vi "Start_Ramping.vi"() -> (3 "Setpoint":dbl)   [LabVIEW 2016]
uses:
  Instrument_Setup.vi
  Global/Global Variables/global.vi
  Global/Global Variables/Data_Display_global.vi
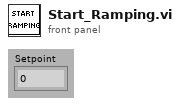
[diagram p1: front panel]
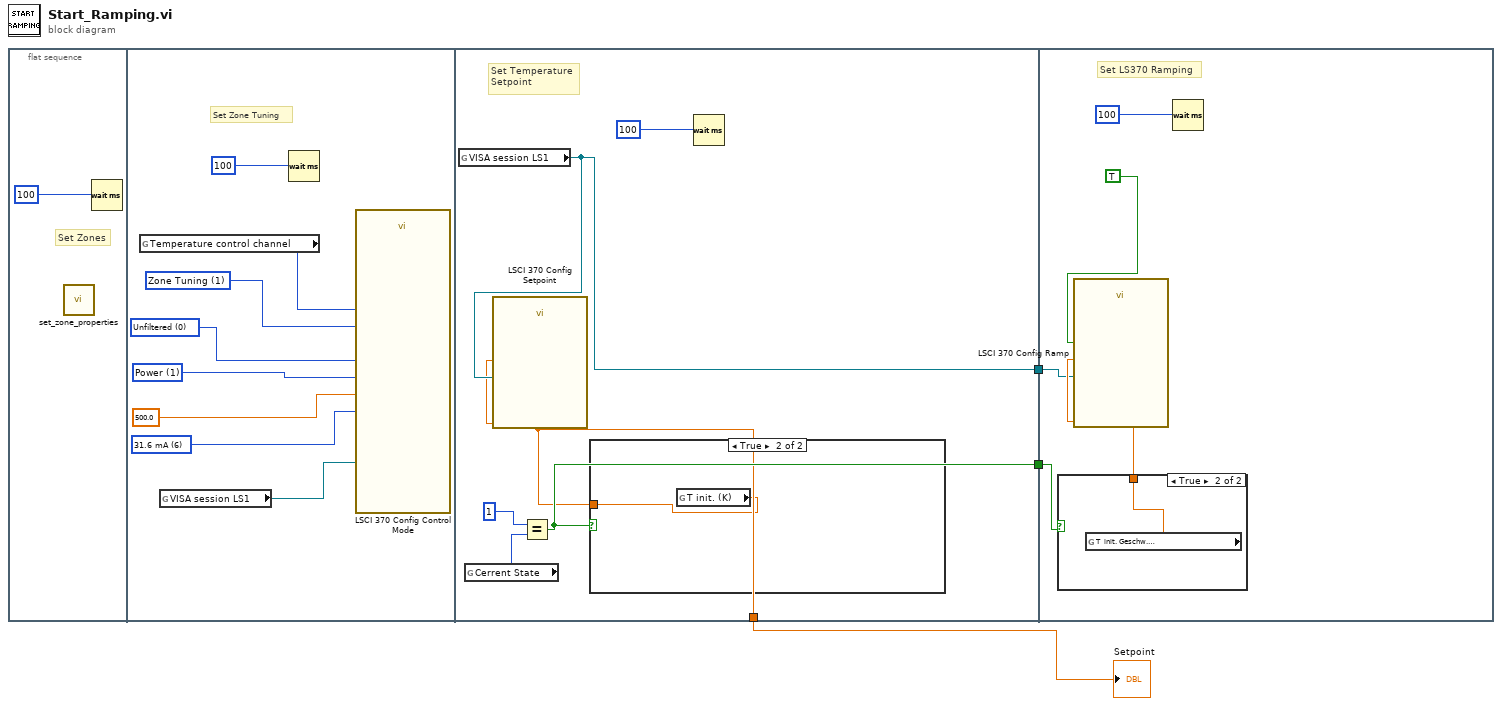
[diagram p0: block diagram]
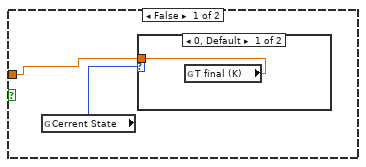
[diagram p2: hidden frame]
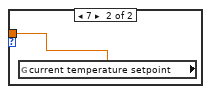
[diagram p3: hidden frame]
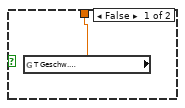
[diagram p4: hidden frame]
diagram:
  n1 = flat-sequence {
    tunnel: [w18] -> w3
    tunnel: [w15] -> w2
    tunnel: [w14] -> w1
    tunnel: w3 -> [w26]
    tunnel: w2 -> [w25]
    frame #0 {
      # "Set Zones"
      n2 = call "set_zone_properties.vi"() -> ()  [unwired: 1 in]
      n3 = Wait (ms)(milliseconds to wait=100) -> ()  [unwired: 1 out]
    }
    frame #1 {
      w11 = u16 6 items=["31.6 uA", "100 uA", "316 uA", "1.00 mA", "3.16 mA", "10.0 mA", "31.6 mA", "100 mA"] ("Maximum Heater Range (0: 31.6 uA)")
      w9 = u16 1 items=["Current", "Power"] ("Heater Output Display (0: Current)")
      w8 = u16 0 items=["Unfiltered", "Filtered"] ("Filtered Readings (0: Unfiltered)")
      w7 = u16 1 items=["Closed Loop PID", "Zone Tuning", "Open Loop", "Off"] ("Control Mode (0: Closed Loop PID)")
      # "Set Zone Tuning"
      n4 = global read "Instrument_Setup.vi" "Temperature control channel"() -> (w6:i32)
      n5 = global read "Instrument_Setup.vi" "VISA session LS1"() -> (w12:refnum<visa-resource-name>)
      n6 = Wait (ms)(milliseconds to wait=100) -> ()  [unwired: 1 out]
      n7 = call "LSCI 370 Config Control Mode.vi"("VISA session"=w12, "Control Mode (0: Closed Loop PID)"=w7, "Channel (1)"=w6, "Filtered Readings (0: Unfiltered)"=w8, "Heater Output Display (0: Current)"=w9, "Heater Resistance (100.00)"=500.0, "Maximum Heater Range (0: 31.6 uA)"=w11) -> ()  [unwired: 7 in, 2 out]
    }
    frame #2 {
      # "Set Temperature\nSetpoint"
      n8 = global read "Instrument_Setup.vi" "VISA session LS1"() -> (w18:refnum<visa-resource-name>)
      n9 = global read "global.vi" "Cerrent State"() -> (w16:i32)
      n10 = Equal?(x=1, y=w16) -> (x = y?=w15:bool)
      n11 = case shown="True" w15 {
        tunnel: [w19 w23] -> w14
        frame False {
          n12 = global read "global.vi" "Cerrent State"() -> (w20:i32)
          n13 = case shown="0, Default" w20 {
            tunnel: [w21 w22] -> w19
            frame 0, Default {
              n14 = global read "global.vi" "T final (K)"() -> (w21:dbl)
            }
            frame 7 {
              n15 = global read "Data_Display_global.vi" "current temperature setpoint"() -> (w22:dbl)
            }
          }
        }
        frame True {
          n16 = global read "global.vi" "T init. (K)"() -> (w23:dbl)
        }
      }
      n17 = call "LSCI 370 Config Setpoint.vi"("VISA session"=w18, "Setpoint (0.00000E+0)"=w14) -> ()  [unwired: 12 in, 2 out]
      n18 = Wait (ms)(milliseconds to wait=100) -> ()  [unwired: 1 out]
    }
    frame #3 {
      # "Set LS370 Ramping"
      n19 = case shown="True" w25 {
        tunnel: [w29 w30] -> w28
        frame False {
          n20 = global read "global.vi" "T Geschw. \n(K/min)"() -> (w29:dbl)
        }
        frame True {
          n21 = global read "global.vi" "T  init. Geschw. \n(K/min)"() -> (w30:dbl)
        }
      }
      n22 = call "LSCI 370 Config Ramp.vi"("VISA session"=w26, "Rate Value (0.001)"=w28, "Ramping On/Off (F: Ramping Off)"=TRUE) -> ()  [unwired: 11 in, 2 out]
      n23 = Wait (ms)(milliseconds to wait=100) -> ()  [unwired: 1 out]
    }
  }
  "Setpoint" <- w1
